vi "2400_4probesweep V2 8Nov.vi"() -> ()   [LabVIEW 2021]
uses:
  <instrlib>/Keithley 24XX/Public/Data/Read (Multiple Points).vi
  <instrlib>/Keithley 24XX/Keithley 24XX.lvlib
  <vilib>/Analysis/NI_AALPro.lvlib
panel:
  in  "Settling delay":dbl=1.0
  in  "Sweep Spacing (0) Linear":u32=5
  out "New file path":path
  in  "Folder to save file to":path
  out "XY Graph":T1(graph)
  out "Intercept":dbl
  out "Slope":dbl
  out "error out":errorcluster
  in  "Source Mode  (0: Voltage)":u16(ring) items=["Voltage", "Current"]
  in  "Number of Points (5)":u32=5
  in  "Timeout (10000 ms)":i32=10000 format="%#.6g"
  in  "Maximum Amplitude (2)":dbl=2.0
  in  "Minimum Amplitude (1)":dbl=1.0
  in  "Compliance  Level (0.1)":dbl=0.1
  in  "Serial Configuration":T2={"Baud Rate"=9600, "Parity"=0, "Data Bits"=8, "Stop Bits"=10, "Flow Control"=0} {"Flow Control" items=["None", "XON/XOFF", "RTS/CTS", "XON/XOFF & RTS/CTS", "DTR/DSR", "XON/XOFF & DTR/DSR"]; "Stop Bits" items=["1.0"=10, "1.5"=15, "2.0"=20]; "Data Bits" items=["7"=7, "8"=8]; "Parity" items=["None", "Odd", "Even", "Mark", "Space"]; "Baud Rate" items=["300"=300, "600"=600, "1200"=1200, "2400"=2400, "4800"=4800, "9600"=9600, "19200"=19200]}
  in  "VISA resource name":refnum<visa-resource-name>
  # "Tested current up to 0.01Amps"
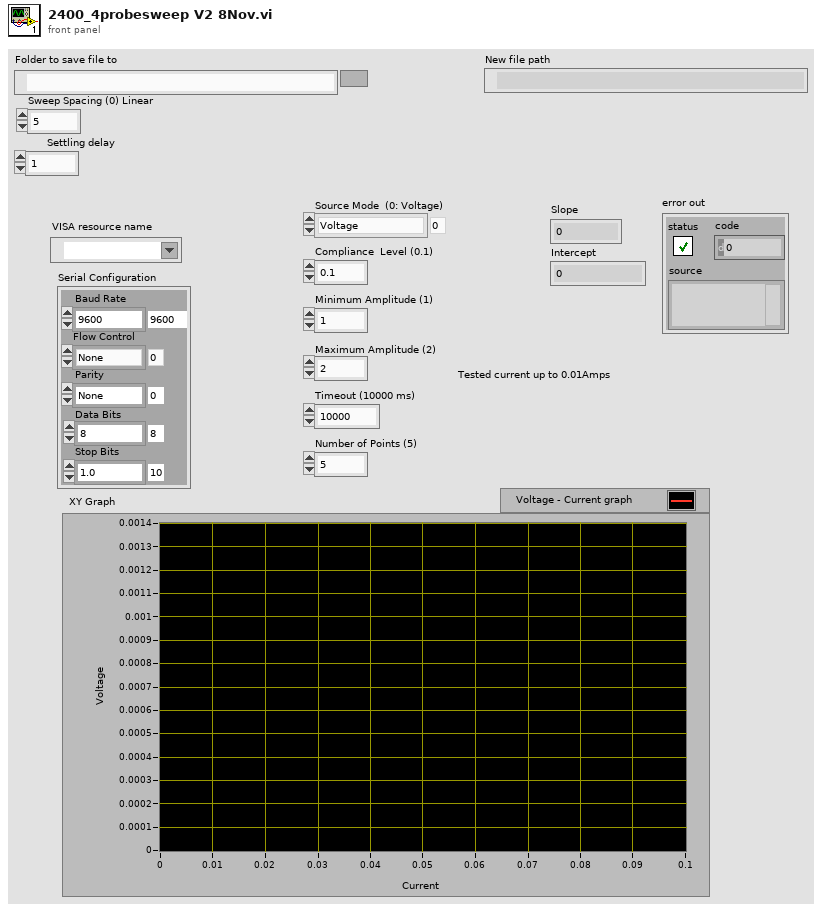
[diagram p1: front panel]
types:
  T1 = cluster{"Current":sgl[], "Best Linear Fit":dbl[]}[]
  T2 = cluster{"Baud Rate":u32, "Parity":u16, "Data Bits":u16, "Stop Bits":u16, "Flow Control":u16}
  T3 = enum16{"open", "replace", "create", "open or create", "replace or create", "replace or create with confirmation"}
  T4 = cluster{"Current":sgl[], "Best Linear Fit":dbl[]}
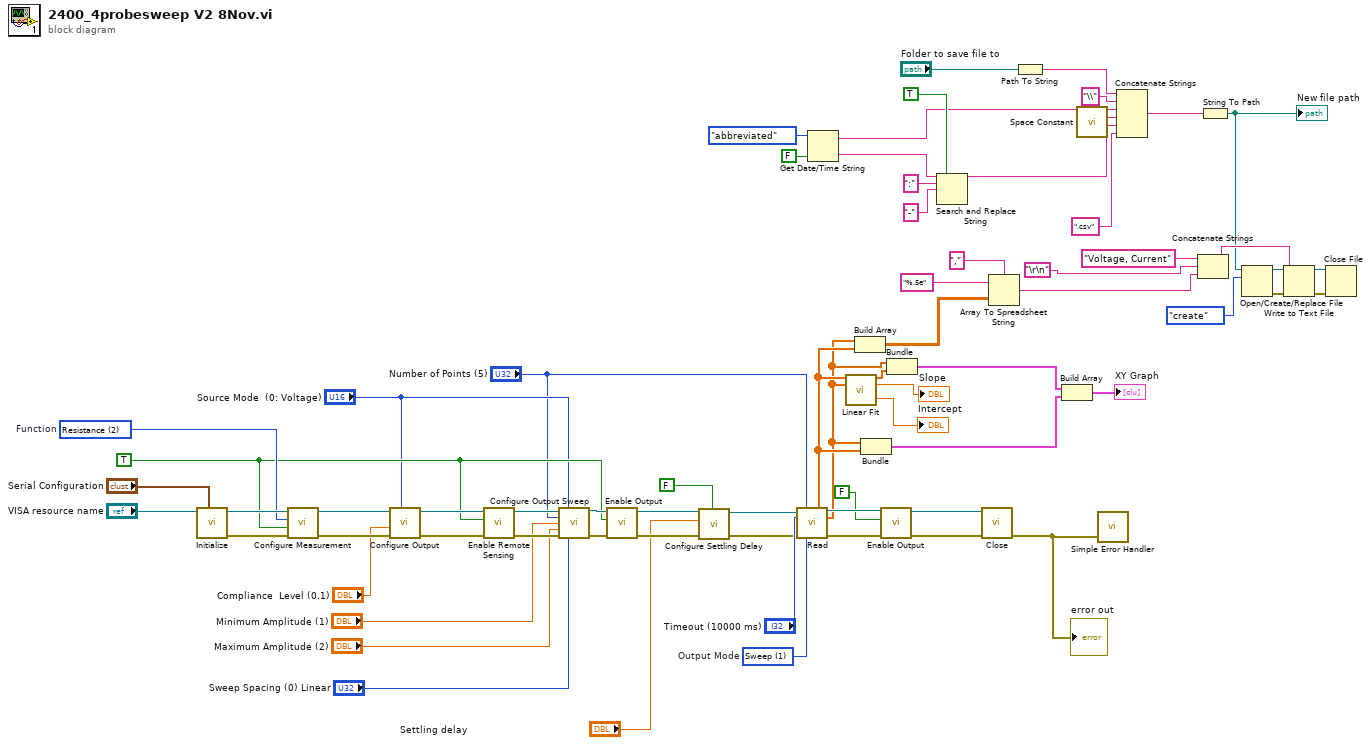
[diagram p0: block diagram]
diagram:
  w47 = u16 1 items=["Fixed", "Sweep", "List"]  # Output Mode
  w53 = u16 2 items=["Volts", "Current", "Resistance"]  # Function
  w52 = TRUE
  n1 = call <instrlib>:"Initialize.vi"("Serial Configuration"="Serial Configuration", "VISA resource name"="VISA resource name") -> ("error out"=w69:errorcluster, "VISA resource name out"=w62:refnum<visa-resource-name>)  [unwired: 8 in]
  n2 = call <instrlib>:"Configure Measurement.vi"("error in (no error)"=w69, "Enable Auto Range (T:Enable)"=w52, "Function (0: Volts)"=w53, "VISA resource name"=w62) -> ("error out"=w68:errorcluster, "VISA resource name out"=w61:refnum<visa-resource-name>)  [unwired: 6 in]
  n3 = call <instrlib>:"Configure Output.vi"("Source Mode  (0: Voltage)"="Source Mode  (0: Voltage)", "error in (no error)"=w68, "Compliance  Level (0.1)"="Compliance  Level (0.1)", "VISA resource name"=w61) -> ("error out"=w67:errorcluster, "VISA resource name out"=w60:refnum<visa-resource-name>)  [unwired: 6 in]
  n4 = call <instrlib>:"Enable Remote Sensing.vi"("error in (no error)"=w67, "Enable Remote Sensing (T: Enable)"=w52, "VISA resource name"=w60) -> ("error out"=w66:errorcluster, "VISA resource name out"=w59:refnum<visa-resource-name>)  [unwired: 7 in]
  n5 = call <instrlib>:"Configure Output Sweep.vi"("VISA resource name"=w59, "Source Mode  (0: Voltage)"="Source Mode  (0: Voltage)", "Number of Points (5)"="Number of Points (5)", "Minimum Amplitude (1)"="Minimum Amplitude (1)", "Maximum Amplitude (2)"="Maximum Amplitude (2)", "error in (no error)"=w66, "Sweep Spacing  (0: Linear)"="Sweep Spacing (0) Linear") -> ("VISA resource name out"=w58:refnum<visa-resource-name>, "error out"=w65:errorcluster)  [unwired: 7 in]
  n6 = call <instrlib>:"Enable Output.vi"("error in (no error)"=w65, "Enable Output (T: Enable)"=w52, "VISA resource name"=w58) -> ("error out"=w6:errorcluster, "VISA resource name out"=w4:refnum<visa-resource-name>)  [unwired: 7 in]
  n7 = call <instrlib>:"Configure Settling Delay.vi"("Auto Settle (T: Enable)"=FALSE, "error in (no error)"=w6, "Manual Settling Delay (0 sec)"="Settling delay", "VISA resource name"=w4) -> ("error out"=w5:errorcluster, "VISA resource name out"=w3:refnum<visa-resource-name>)  [unwired: 6 in]
  n8 = call-poly <instrlib>:"Read.vi"("VISA resource name"=w3, "Sample Count (1)"="Number of Points (5)", "Timeout (10000 ms)"="Timeout (10000 ms)", "error in (no error)"=w5, "Output Mode (0: Fixed)"=w47) -> ("Voltage"=w36:sgl[], "VISA resource name out"=w57:refnum<visa-resource-name>, "Current"=w35:sgl[], "error out"=w64:errorcluster)  [unwired: 4 in, 3 out]
  n9 = Get Date/Time String(date format (0)=enum16{"short", "long", "abbreviated"}."abbreviated", want seconds? (F)=FALSE) -> (date string=w22:string, time string=w25:string)  [unwired: 1 in]
  n10 = call <vilib>:"Linear Fit.vi"("Y"=w36, "X"=w35) -> ("Best Linear Fit"=w39:dbl[], "slope"=→"Slope":dbl, "intercept"=→"Intercept":dbl)  [unwired: 9 in, 2 out]
  n11 = Build Array(w35, w36) -> (w34:sgl[][])
  n12 = Bundle("Current"=w35, "Voltage"=w36) -> (w37:cluster{"Current":sgl[], "Voltage":sgl[]})  [unwired: 1 in]
  n13 = call <instrlib>:"Enable Output.vi"("error in (no error)"=w64, "Enable Output (T: Enable)"=FALSE, "VISA resource name"=w57) -> ("error out"=w63:errorcluster, "VISA resource name out"=w56:refnum<visa-resource-name>)  [unwired: 7 in]
  n14 = Bundle("Current"=w35, "Best Linear Fit"=w39) -> (w38:T4)  [unwired: 1 in]
  n15 = Search and Replace String(replace all?=TRUE ("replace all? (F)"), input string=w25, search string=":" ("replace string (\"\")"), replace string="-" ("replace string (\"\")")) -> (result string=w20:string)  [unwired: 4 in, 3 out]
  n16 = call <instrlib>:"Close.vi"("error in (no error)"=w63, "VISA resource name"=w56) -> ("error out"=w43:errorcluster)  [unwired: 9 in]
  "error out" <- w43
  n17 = Array To Spreadsheet String(delimiter (Tab)=",", array=w34, 3:"%.5e") -> (spreadsheet string=w32:string)
  n18 = Path To String(path="Folder to save file to") -> (string=w16:string)
  n19 = Build Array(w38, w37) -> (→"XY Graph":T1)
  n20 = call <vilib>:"Space Constant.vi"() -> ("String"=w21:string)
  n21 = call <vilib>:"Simple Error Handler.vi"("error in (no error)"=w43) -> ()  [unwired: 4 in, 5 out]
  n22 = Concatenate Strings "Concatenate Strings"(w16, "\\" ("string"), w22, w21, w20, ".csv" ("string")) -> (w18:string)
  n23 = Concatenate Strings("Voltage, Current", "\r\n", w32) -> (w28:string)
  n24 = String To Path(string=w18) -> (path=w11:path)
  "New file path" <- w11
  n25 = Open/Create/Replace File(file path (use dialog)=w11, operation (0:open)=T3."create") -> (refnum out=w10:refnum<file>, error out=w9:errorcluster)  [unwired: 4 in, 1 out]
  n26 = Write to Text File(file (use dialog)=w10, text=w28, error in=w9) -> (refnum out=w13:refnum<file>, error out=w12:errorcluster)  [unwired: 1 in, 1 out]
  n27 = Close File(refnum=w13, error in=w12) -> ()  [unwired: 2 out]
